vi "test Init OD Entry_1.vi"(11 "Test Case In":refnum<class "test EDS.lvclass">) -> (0 "error out":errorcluster, 3 "Test Case Out":refnum<class "test EDS.lvclass">)   [LabVIEW 2024]
uses:
  test EDS.lvclass
  C:/Program Files/National Instruments/LabVIEW 2024/vi.lib/Astemes/LUnit/Test Case.lvclass
  Core/EDS/EDS.lvclass
  Core/Object Type.ctl
  Core/Data Type.ctl
  Core/Access Type.ctl
  Core/EDS/EDS.lvclass/EDS.ctl
  <vilib>/Astemes/LUnit/Test Case.lvclass/Test Case.ctl
  <vilib>/Astemes/LUnit/Append Fail Result.vi
  <vilib>/Astemes/LUnit/Append Pass Result.vi
  <vilib>/Astemes/LUnit/Run In UI.vi
  <vilib>/Utility/error.llb/Clear Errors.vi
  Core/OD Sub-Entry/OD Sub-Entry.lvclass
  D:/git/EDS-File-Viewer/Core/OD Entry/OD Entry.lvclass
  Core/Sorted Object Dictionary/Sorted Object Dictionary.lvclass
  Core/OD Entry/OD Entry.lvclass
  <vilib>/Astemes/LUnit/Test Case.lvclass
  Core/EDS.lvlib
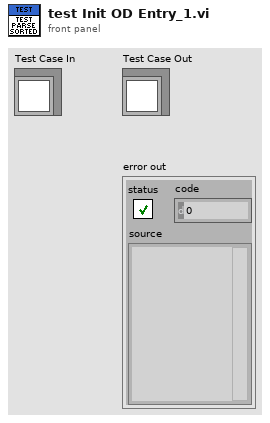
[diagram p1: front panel]
types:
  T1 = typedef "EDS.lvlib/Access Type.ctl" = enum16{"rw", "ro", "wo", "rwr", "rww", "const"}
  T2 = typedef "EDS.lvlib/Data Type.ctl" = u16
  T3 = typedef "EDS.lvlib/Object Type.ctl" = u8
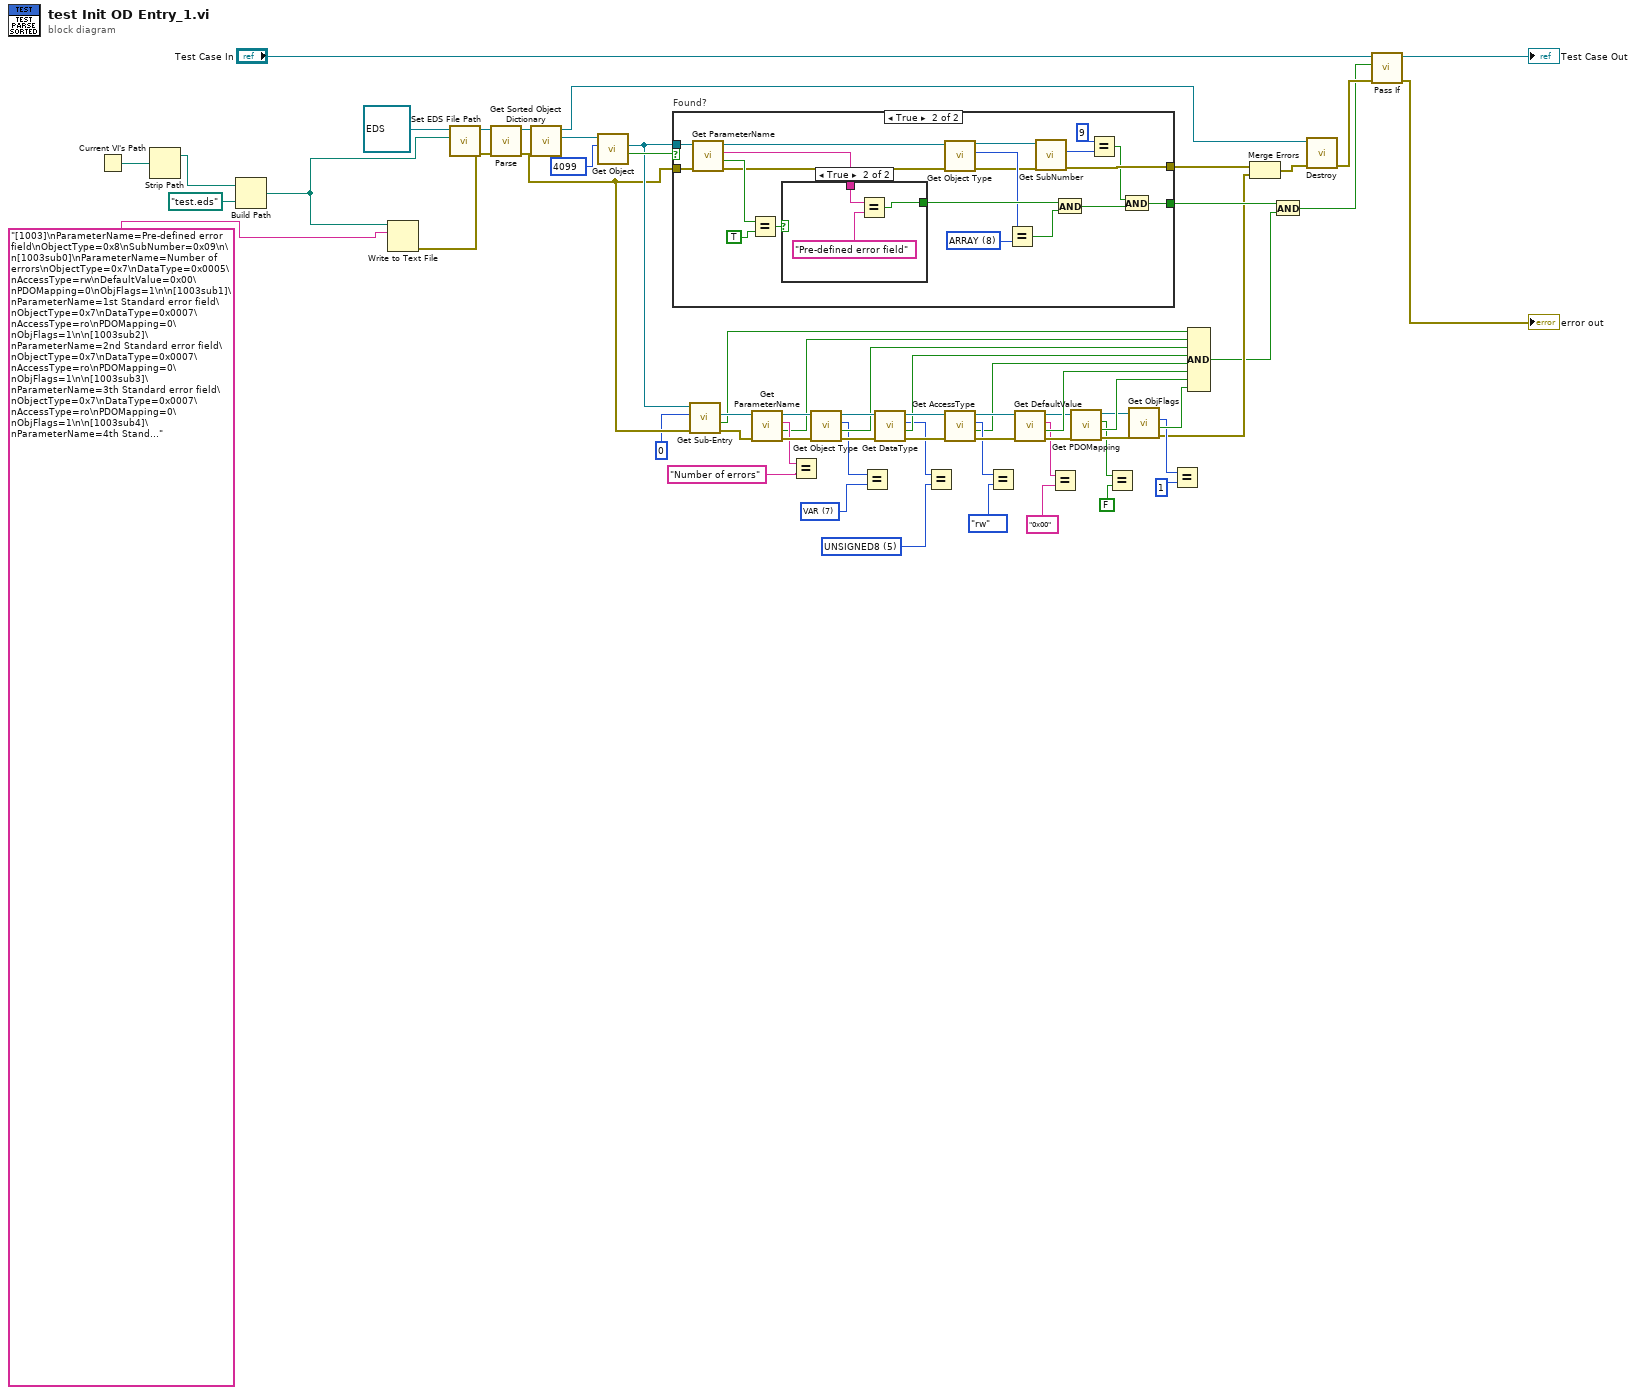
[diagram p0: block diagram]
diagram:
  w21 = T2 5 items=["BOOLEAN"=1, "INTEGER8"=2, "INTEGER16"=3, "INTEGER32"=4, "UNSIGNED8"=5, "UNSIGNED16"=6, "UNSIGNED32"=7, "REAL32"=8, "VISIBLE_STRING"=9, "OCTET_STRING"=10, "UNICODE_STRING"=11, "TIME_OF_DAY"=12, "TIME_DIFFERENCE"=13, "RESERVED1"=14, "DOMAIN"=15, "INTEGER24"=16, "REAL64"=17, "INTEGER40"=18, "INTEGER48"=19, "INTEGER56"=20, "INTEGER64"=21, "UNSIGNED24"=22, "RESERVED2"=23, "UNSIGNED40"=24, "UNSIGNED48"=25, "UNSIGNED56"=26, "UNSIGNED64"=27, "RESERVED3"=28, "RESERVED4"=29, "RESERVED5"=30, "RESERVED6"=31, "PDO_COMMUNICATION_PARAMETER"=32, "PDO_MAPPING"=33, "SDO_PARAMETER"=34, "IDENTITY"=35, "RESERVED7"=36] ("DataType")
  w23 = T3 7 items=["NULL"=0, "DOMAIN"=2, "DEFTYPE"=5, "DEFSTRUCT"=6, "VAR"=7, "ARRAY"=8, "RECORD"=9] ("ObjectType")
  n1 = Current VI's Path() -> (path=w57:path)
  n2 = Strip Path(path=w57) -> (stripped path=w53:path)  [unwired: 1 out]
  n3 = Build Path(base path=w53, name or relative path=path "test.eds") -> (appended path=w54:path)
  n4 = Write to Text File(file (use dialog)=w54, text="[1003]\nParameterName=Pre-defined error field\nObjectType=0x8\nSubNumber=0x09\n\n[1003sub0]\nParameterName=Number of errors\nObjectType=0x7\nDataType=0x0005\nAccessType=rw\nDefaultValue=0x00\nPDOMapping=0\nObjFlags=1\n\n[1003sub1]\nParameterName=1st Standard error field\nObjectType=0x7\nDataType=0x0007\nAccessType=ro\nPDOMapping=0\nObjFlags=1\n\n[1003sub2]\nParameterName=2nd Standard error field\nObjectType=0x7\nDataType=0x0007\nAccessType=ro\nPDOMapping=0\nObjFlags=1\n\n[1003sub3]\nParameterName=3th Standard error field\nObjectType=0x7\nDataType=0x0007\nAccessType=ro\nPDOMapping=0\nObjFlags=1\n\n[1003sub4]\nParameterName=4th Standard error field\nObjectType=0x7\nDataType=0x0007\nAccessType=ro\nPDOMapping=0\nObjFlags=1\n\n[1003sub5]\nParameterName=5th Standard error field\nObjectType=0x7\nDataType=0x0007\nAccessType=ro\nPDOMapping=0\nObjFlags=1\n\n[1003sub6]\nParameterName=6th Standard error field\nObjectType=0x7\nDataType=0x0007\nAccessType=ro\nPDOMapping=0\nObjFlags=1\n\n[1003sub7]\nParameterName=7th Standard error field\nObjectType=0x7\nDataType=0x0007\nAccessType=ro\nPDOMapping=0\nObjFlags=1\n\n[1003sub8]\nParameterName=8th Standard error field\nObjectType=0x7\nDataType=0x0007\nAccessType=ro\nPDOMapping=0\nObjFlags=1") -> (error out=w55:errorcluster)  [unwired: 2 in, 2 out]
  n5 = call "Set EDS File Path.vi"("EDS File Path"=w54, "EDS in"=refnum<class "EDS.lvclass"> refnum ("EDS.lvlib:EDS.lvclass")) -> ("EDS out"=w58:refnum<class "EDS.lvclass">)  [unwired: 9 in]
  n6 = call "Parse.vi"("error in"=w55, "EDS in"=w58) -> ("error out"=w42:errorcluster, "EDS out"=w52:refnum<class "EDS.lvclass">)  [unwired: 8 in]
  n7 = call "Get Sorted Object Dictionary.vi"("EDS in"=w52) -> ("Sorted Object Dictionary"=w49:refnum<class "Sorted Object Dictionary.lvclass">, "EDS out"=w51:refnum<class "EDS.lvclass">)  [unwired: 9 in]
  n8 = call "Get Object.vi"("Numeric"=u16 4099, "Sorted Object Dictionary in"=w49) -> ("Found?"=w44:bool, "OD Entry"=w43:refnum<class "OD Entry.lvclass">)  [unwired: 7 in, 1 out]
  n9 = case "Found?" shown="True" w44 {
    selector: w44 -> [w63 _]
    tunnel: w43 -> [_ w84]
    tunnel: w42 -> [w64 w83]
    tunnel: [w63 w66] -> w47
    tunnel: [w64 w70] -> w45
    frame False {
    }
    frame True {
      w74 = T3 8 items=["NULL"=0, "DOMAIN"=2, "DEFTYPE"=5, "DEFSTRUCT"=6, "VAR"=7, "ARRAY"=8, "RECORD"=9] ("y")
      n10 = call "Get ParameterName.vi"("Error In"=w83, "reference in"=w84) -> ("Error Out"=w76:errorcluster, "Defined?"=w82:bool, "ParameterName"=w80:string, "reference out"=w77:refnum<class "OD Entry.lvclass">)  [unwired: 6 in]
      n11 = Equal?(x=w82, y=TRUE) -> (x = y?=w79:bool)
      n12 = case shown="True" w79 {
        selector: w79 -> [w85 _]
        tunnel: w80 -> [_ w88]
        tunnel: [w85 w86] -> w78
        frame False {
        }
        frame True {
          n13 = Equal?(x=w88, y="Pre-defined error field") -> (x = y?=w86:bool)
        }
      }
      n14 = call "Get Object Type.vi"("Error In"=w76, "reference in"=w77) -> ("Error Out"=w71:errorcluster, "ObjectType"=w75:T3, "reference out"=w69:refnum<class "OD Entry.lvclass">)  [unwired: 6 in, 1 out]
      n15 = Equal?(x=w75, y=w74) -> (x = y?=w72:bool)
      n16 = call "Get SubNumber.vi"("Error In"=w71, "reference in"=w69) -> ("Error Out"=w70:errorcluster, "SubNumber"=w68:u8)  [unwired: 6 in, 2 out]
      n17 = And(x=w78, y=w72) -> (x .and. y?=w73:bool)
      n18 = Equal?(x=u8 9, y=w68) -> (x = y?=w65:bool)
      n19 = And(x=w65, y=w73) -> (x .and. y?=w66:bool)
    }
  }
  n20 = call "Get Sub-Entry.vi"("Error In"=w42, "Sub-Index"=u16 0, "reference in"=w43) -> ("Error Out"=w40:errorcluster, "Found?"=w28:bool, "OD Sub-Entry"=w41:refnum<class "OD Sub-Entry.lvclass">)  [unwired: 5 in, 1 out]
  n21 = call "Get ParameterName.vi"("Error In"=w40, "reference in"=w41) -> ("Error Out"=w39:errorcluster, "Defined?"=w27:bool, "ParameterName"=w30:string, "reference out"=w38:refnum<class "OD Sub-Entry.lvclass">)  [unwired: 6 in]
  n22 = Equal?(x=w30, y="Number of errors") -> ()  [unwired: 1 out]
  n23 = call "Get Object Type.vi"("Error In"=w39, "reference in"=w38) -> ("Error Out"=w36:errorcluster, "Defined?"=w26:bool, "ObjectType"=w24:T3, "reference out"=w37:refnum<class "OD Sub-Entry.lvclass">)  [unwired: 6 in]
  n24 = Equal?(x=w24, y=w23) -> ()  [unwired: 1 out]
  n25 = call "Get DataType.vi"("Error In"=w36, "reference in"=w37) -> ("Error Out"=w33:errorcluster, "Set?"=w25:bool, "DataType"=w22:T2, "reference out"=w34:refnum<class "OD Sub-Entry.lvclass">)  [unwired: 6 in]
  n26 = Equal?(x=w22, y=w21) -> ()  [unwired: 1 out]
  n27 = call "Get AccessType.vi"("Error In"=w33, "reference in"=w34) -> ("Error Out"=w31:errorcluster, "Defined?"=w18:bool, "AccessType"=w20:T1, "reference out"=w32:refnum<class "OD Sub-Entry.lvclass">)  [unwired: 6 in]
  n28 = Equal?(x=w20, y=Access_Type."rw") -> ()  [unwired: 1 out]
  n29 = call "Get DefaultValue.vi"("Error In"=w31, "reference in"=w32) -> ("Error Out"=w14:errorcluster, "Set?"=w17:bool, "DefaultValue"=w10:string, "reference out"=w15:refnum<class "OD Sub-Entry.lvclass">)  [unwired: 6 in]
  n30 = Equal?(x=w10, y="0x00") -> ()  [unwired: 1 out]
  n31 = call "Get PDOMapping.vi"("Error In"=w14, "reference in"=w15) -> ("Error Out"=w12:errorcluster, "Defined?"=w16:bool, "PDOMapping"=w8:bool, "reference out"=w13:refnum<class "OD Sub-Entry.lvclass">)  [unwired: 6 in]
  n32 = Equal?(x=w8, y=FALSE) -> ()  [unwired: 1 out]
  n33 = call "Get ObjFlags.vi"("Error In"=w12, "reference in"=w13) -> ("Error Out"=w4:errorcluster, "Defined?"=w11:bool, "ObjFlags"=w6:u32)  [unwired: 6 in, 1 out]
  n34 = Equal?(x=w6, y=u32 1) -> ()  [unwired: 1 out]
  n35 = Compound Arithmetic op=AND(w28, w27, w26, w25, w18, w17, w16, w11) -> (w2:bool)
  n36 = Merge Errors(w45, w4) -> (w5:errorcluster)
  n37 = And(x=w47, y=w2) -> (x .and. y?=w3:bool)
  n38 = call "Destroy.vi"("error in"=w5, "EDS in"=w51) -> ("error out"=w46:errorcluster)  [unwired: 8 in, 1 out]
  n39 = call <vilib>:"Pass If.vi"("error in (no error)"=w46, "Pass?"=w3, "LUnit Test Case In"="Test Case In") -> ("error out"=→"error out":errorcluster, "LUnit Test Case Out"=→"Test Case Out":refnum<class "test EDS.lvclass">)  [unwired: 7 in]
